vi "Ports To System Definition.vi"(8 "error in":errorcluster, 9 "ports":T2[](array[typedef]), 10 "parameter configuration file path":path, 11 "custom device ref":T1 format="%.0x") -> (0 "error out":errorcluster, 3 "custom device ref out":T1 format="%.0x")   [LabVIEW 2020, in "Ballard ARINC 429 Scripting.lvlib"]
uses:
  Ballard ARINC 429 Scripting.lvlib
  <vilib>/NI VeriStand/Custom Device API/Custom Device Item Ref.ctl
  Shared/VS Channels Definition for All Labels on Hardware Channel.ctl
  Shared/VS Channels Definition for Label.ctl
  Shared/VS Channel Definition for Parameter.ctl
  Shared/Direction.ctl
  Shared/Parameter Definition.ctl
  Encoding and Decoding/Encoding.ctl
  Shared/Transfer Type.ctl
  <vilib>/NI VeriStand/Custom Device API/Custom Device API.lvlib
  Encoding and Decoding/Encoding and Decoding.lvlib
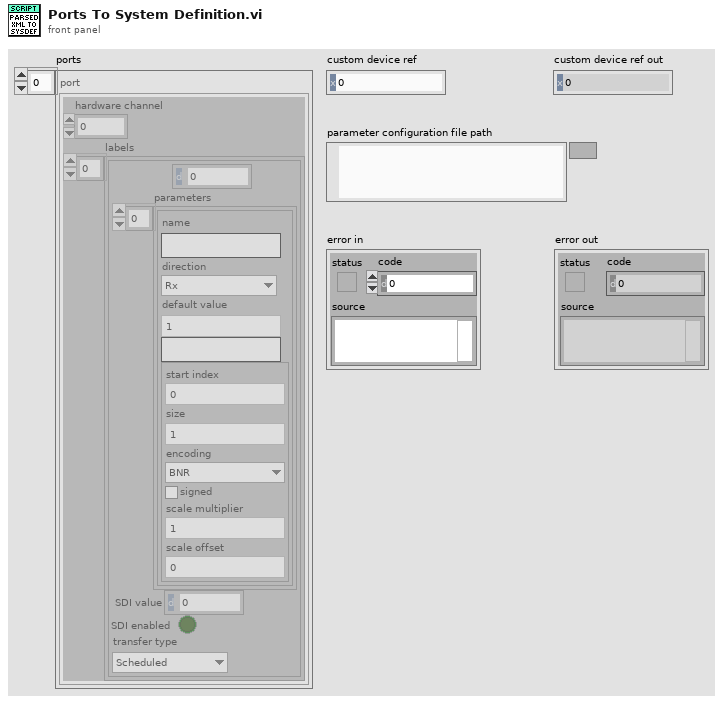
[diagram p1: front panel]
types:
  T1 = typedef "Custom Device API.lvlib/Custom Device Item Ref.ctl" = u64
  T2 = typedef "VS Channels Definition for All Labels on Hardware Channel.ctl" = cluster{"hardware channel":i32, "labels":T3[]}
  T3 = typedef "VS Channels Definition for Label.ctl" = cluster{"label (Dec)":u32, "parameters":T4[], "SDI value":u8, "SDI enabled":bool, "transfer type":T8}
  T4 = typedef "VS Channel Definition for Parameter.ctl" = cluster{"name":string, "direction":T5, "default value":dbl, "unit":string, "Parameter":T6}
  T5 = typedef "Direction.ctl" = enum16{"Rx", "Tx"}
  T6 = typedef "Parameter Definition.ctl" = cluster{"start index":i32, "size":i32, "encoding":T7, "signed":bool, "scale multiplier":dbl, "scale offset":dbl}
  T7 = typedef "Encoding and Decoding.lvlib/Encoding.ctl" = enum16{"BNR", "BCD", "Discrete"}
  T8 = typedef "Transfer Type.ctl" = enum16{"Scheduled", "Acyclic", "Block", "Strobe"}
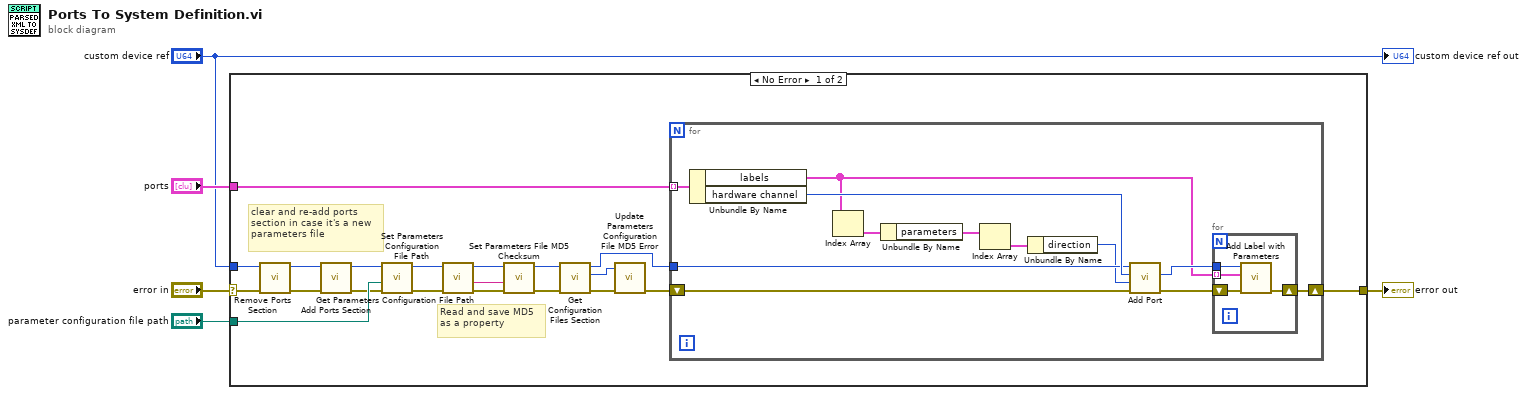
[diagram p0: block diagram]
diagram:
  n1 = case shown="No Error" "error in" {
    selector: "error in" -> [w21 w42]
    tunnel: "custom device ref" -> [w22 _]
    tunnel: [w25 w42] -> w5
    tunnel: "ports" -> [w24 _]
    tunnel: "parameter configuration file path" -> [w23 _]
    frame No Error {
      # "Read and save MD5 as a property"
      # "clear and re-add ports section in case it's a new parameters file"
      n2 = call "Remove Ports Section.vi"("error in"=w21, "custom device ref"=w22) -> ("error out"=w20:errorcluster, "custom device ref out"=w19:T1)  [unwired: 8 in]
      n3 = call "Add Ports Section.vi"("error in"=w20, "custom device ref"=w19) -> ("error out"=w17:errorcluster, "custom device ref out"=w18:T1)  [unwired: 7 in, 1 out]
      n4 = call "Set Parameters Configuration File Path.vi"("error in"=w17, "path"=w23, "custom device ref"=w18) -> ("error out"=w16:errorcluster, "custom device ref out"=w15:T1)  [unwired: 7 in]
      n5 = call "Get Parameters Configuration File Path.vi"("error in"=w16, "custom device ref"=w15) -> ("error out"=w13:errorcluster, "MD5"=w12:string, "custom device ref out"=w14:T1)  [unwired: 6 in, 1 out]
      n6 = call "Set Parameters File MD5 Checksum.vi"("error in"=w13, "MD5"=w12, "custom device ref"=w14) -> ("error out"=w10:errorcluster, "custom device ref out"=w11:T1)  [unwired: 7 in]
      n7 = call "Get Configuration Files Section.vi"("error in"=w10, "Custom device Ref"=w11) -> ("error out"=w9:errorcluster, "Configuration files Ref"=w7:T1, "Custom device Ref out"=w6:T1)  [unwired: 7 in]
      n8 = call "Update Parameters Configuration File MD5 Error.vi"("error in"=w9, "configuration files ref"=w7) -> ("error out"=w8:errorcluster)  [unwired: 8 in, 1 out]
      n9 = for {
        shift-right: [w34] -> w25
        shift-left: w8 -> [w31]
        tunnel: w6 -> [w32]
        tunnel: w24 -> [w37] mode=indexing
        n10 = Unbundle By Name(w37) -> ("labels"=w30:T3[], "hardware channel"=w33:i32)
        n11 = Index Array(array=w30) -> (element=w29:T3)  [unwired: 1 in]
        n12 = Unbundle By Name(w29) -> ("parameters"=w28:T4[])
        n13 = Index Array(array=w28) -> (element=w27:T4)  [unwired: 1 in]
        n14 = Unbundle By Name(w27) -> ("direction"=w26:T5)
        n15 = call "Add Port.vi"("error in"=w31, "direction"=w26, "port number"=w33, "custom device ref"=w32) -> ("error out"=w36:errorcluster, "port ref out"=w35:T1)  [unwired: 5 in, 1 out]
        n16 = for {
          tunnel: w35 -> [w40]
          tunnel: w30 -> [w38] mode=indexing
          shift-right: [w39] -> w34
          shift-left: w36 -> [w41]
          n17 = call "Add Label with Parameters.vi"("error in"=w41, "label"=w38, "port ref"=w40) -> ("error out"=w39:errorcluster)  [unwired: 7 in, 1 out]
        }
      }
    }
    frame Error {
    }
  }
  "error out" <- w5
  "custom device ref out" <- "custom device ref"
